vi "Add Word.vi"(7 "highlight? (F)":bool, 8 "error in":errorcluster, 10 "name (Word)":string="Word", 11 "label ref":T1 format="%.0x") -> (0 "error out":errorcluster, 1 "newly created?":bool, 2 "word ref":T1 format="%.0x", 3 "label ref out":T1 format="%.0x")   [LabVIEW 2020, in "Ballard ARINC 429 Scripting.lvlib"]
uses:
  Ballard ARINC 429 Scripting.lvlib
  <vilib>/NI VeriStand/Custom Device API/Custom Device Item Ref.ctl
  Constants.vi
  <vilib>/NI VeriStand/Custom Device API/Custom Device API.lvlib
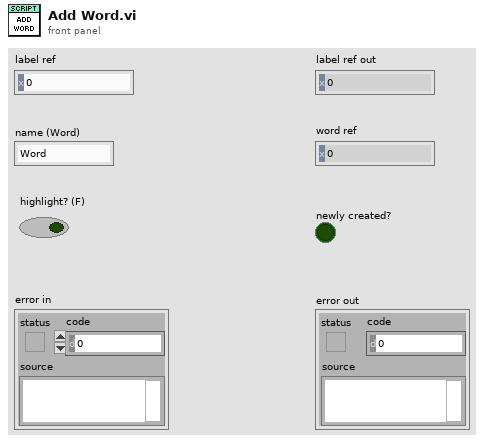
[diagram p1: front panel]
types:
  T1 = typedef "Custom Device API.lvlib/Custom Device Item Ref.ctl" = u64
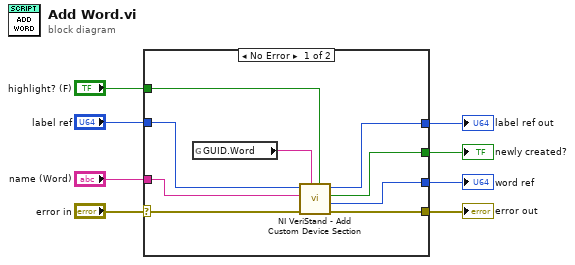
[diagram p0: block diagram]
diagram:
  n1 = case shown="No Error" "error in" {
    selector: "error in" -> [w17 w19]
    tunnel: [w16 w19] -> w7
    tunnel: "label ref" -> [w14 w18]
    tunnel: [w13 _] -> w5
    tunnel: "name (Word)" -> [w15 _]
    tunnel: "highlight? (F)" -> [w12 _]
    tunnel: [w11 _] -> w2
    tunnel: [w10 w18] -> w1
    frame No Error {
      n2 = global read "Constants.vi" "GUID.Word"() -> (w9:string)
      n3 = call <vilib>:"NI VeriStand - Add Custom Device Section.vi"("Highlight? (F)"=w12, "GUID (Default Section)"=w9, "error in (no error)"=w17, "Section Name"=w15, "Parent Ref in"=w14) -> ("error out"=w16:errorcluster, "Section Ptr"=w13:T1, "Newly Created?"=w11:bool, "Parent Ref out"=w10:T1)  [unwired: 3 in]
    }
    frame Error {
    }
  }
  "word ref" <- w5
  "error out" <- w7
  "newly created?" <- w2
  "label ref out" <- w1
